vi "Step4.vi"(1 "U":dbl[][](array[numeric]), 2 "U0":dbl[][](array[numeric]), 3 "n":i32, 4 "j":i32) -> (0 "Numeric":dbl)   [LabVIEW 2011]
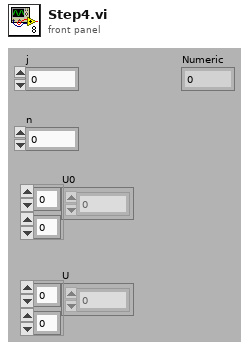
[diagram p1: front panel]
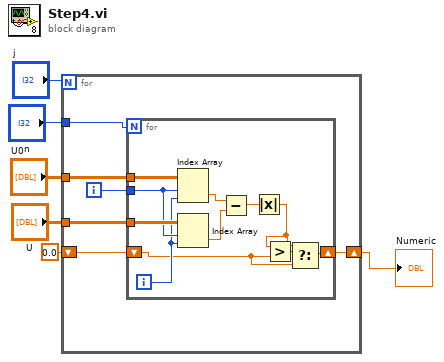
[diagram p0: block diagram]
diagram:
  n1 = for {
    N: "j" -> [_]
    tunnel: "U0" -> [w12]
    tunnel: "U" -> [w11]
    shift-right: [w8] -> w5
    shift-left: 0.0 -> [w9]
    tunnel: "n" -> [w7]
    i -> [w10]
    n2 = for {
      N: w7 -> [_]
      tunnel: w12 -> [w23]
      tunnel: w11 -> [w22]
      tunnel: w10 -> [w21]
      shift-right: [w13] -> w8
      shift-left: w9 -> [w14]
      i -> [w20]
      n3 = Index Array(array=w23, index (row)=w21, index (col)=w20) -> (element=w19:dbl)
      n4 = Index Array(array=w22, index (row)=w21, index (col)=w20) -> (element=w18:dbl)
      n5 = Subtract(x=w19, y=w18) -> (x-y=w17:dbl)
      n6 = Absolute Value(x=w17) -> (abs(x)=w15:dbl)
      n7 = Greater?(x=w15, y=w14) -> (0:w16:bool)
      n8 = Select(t=w15, s=w16, f=w14) -> (s? t:f=w13:dbl)
    }
  }
  "Numeric" <- w5
